vi "DiffDrivePoseEst2_Relative_Example.vi"() -> ()   [LabVIEW 2019]
doc: "This WebSockets API example VI acts as a server for an incoming websockets connection. Receives/sends string data to the connected client."
uses:
  <vilib>/Rock Robotics/WPI/ThirdParty/JAS_Junk/TrajLib/Trajectory_Library.lvlib
  <vilib>/Rock Robotics/WPI/ThirdParty/JAS_Junk/TrajLib/TypeDef/FieldDisp_ElementPicture.ctl
  <vilib>/Rock Robotics/WPI/ThirdParty/JAS_Junk/TrajLib/TypeDef/TRANSLATION2D.ctl
  <vilib>/Rock Robotics/WPI/ThirdParty/JAS_Junk/TrajLib/TypeDef/ROTATION2D.ctl
  <vilib>/Rock Robotics/WPI/ThirdParty/JAS_Junk/TrajLib/TypeDef/POSE2D.ctl
panel:
  in  "Ramsette\nAuto":bool=TRUE
  out "Odom Pose\n Ft, Deg":T1 {"ROTATION"."SIN" format="%13.4f"; "ROTATION"."COS" format="%13.4f"; "ROTATION"."VALUE" format="%13.4f"; "TRANSLATION"."Y" format="%14.3f"; "TRANSLATION"."X" format="%14.3f"}
  out "Trajectory\nAtReference":bool
  out "ROBOT":T4
  in  "Tab Control":T5(tab)
  out "Field Picture":picture
  out "Right Motor Dmd":dbl format="%20.3f"
  out "Left Motor Dmd":dbl format="%20.3f"
  out "Gyro Heading (Deg)":dbl format="%20.3f"
  out "Left Motor Dist (Ft)":dbl format="%20.3f"
  out "Right Motor Dist (Ft)":dbl format="%20.3f"
  out "Left Motor Vel - PV (Ft/Sec)":dbl format="%20.3f"
  out "Right Motor Vel - PV (Ft/Sec)":dbl format="%20.3f"
  out "Odometry sim abs\n Pose":T1={"TRANSLATION"={"X"=1.0, "Y"=1.0}, "ROTATION"={"VALUE"=0.0, "COS"=1.0, "SIN"=0.0}} {"ROTATION"."SIN" format="%13.4f"; "ROTATION"."COS" format="%13.4f"; "ROTATION"."VALUE" format="%13.4f"; "TRANSLATION"."Y" format="%14.3f"; "TRANSLATION"."X" format="%14.3f"}
  out "Trajectory Error":T6(graph)
  in  "Follow Relative\nTrajectory":bool
  in  "Spin Right":bool
  in  "Spin Left":bool
  in  "Reverse":bool
  in  "Forward":bool
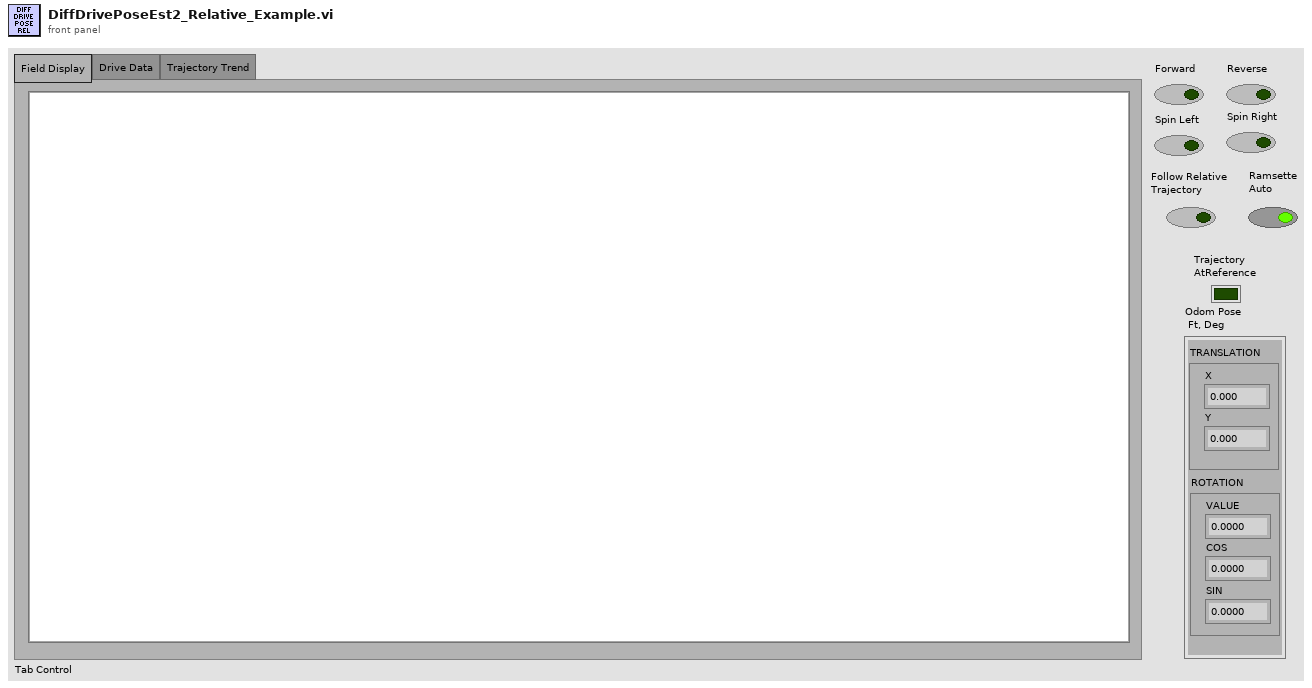
[diagram p1: front panel]
types:
  T1 = typedef "Trajectory_Library.lvlib/POSE2D.ctl" = cluster{"TRANSLATION":T2, "ROTATION":T3}
  T2 = typedef "Trajectory_Library.lvlib/TRANSLATION2D.ctl" = cluster{"X":dbl, "Y":dbl}
  T3 = typedef "Trajectory_Library.lvlib/ROTATION2D.ctl" = cluster{"VALUE":dbl, "COS":dbl, "SIN":dbl}
  T4 = typedef "Trajectory_Library.lvlib/FieldDisp_ElementPicture.ctl" = picture
  T5 = enum32{"Field Display", "Drive Data", "Trajectory Trend"}
  T6 = cluster{"Traj X Err Ft":dbl, "Traj Y Err Ft":dbl, "Traj Heading Err Deg":dbl, dbl}
  T7 = typedef "Trajectory_Library.lvlib/FieldDisp_FieldElement.ctl" = cluster{"ONE-8-bit pixmap":u8[][], "Two-Array":cdb[][], "Three-Numeric":i32, "Four-Numeric":i32, "Five-Numeric":cdb, "Six-colors":u32[], "Seven-new element/subarray":u32, "Left Poxel":dbl, "Top Pixel":dbl, "Width Pix/Ft":dbl, "Height Pix/Ft":dbl, "Element Picture Ref":refnum<vi>}
  T8 = typedef "Trajectory_Library.lvlib/TRAJECTORY.ctl" = cluster{"TotalTImeSecs":dbl, "States":T9[]}
  T9 = typedef "Trajectory_Library.lvlib/TRAJ_STATE.ctl" = cluster{"TimeSeconds":dbl, "Velocity":dbl, "Acceleration":dbl, "POSE":T1, "Curvature":dbl}
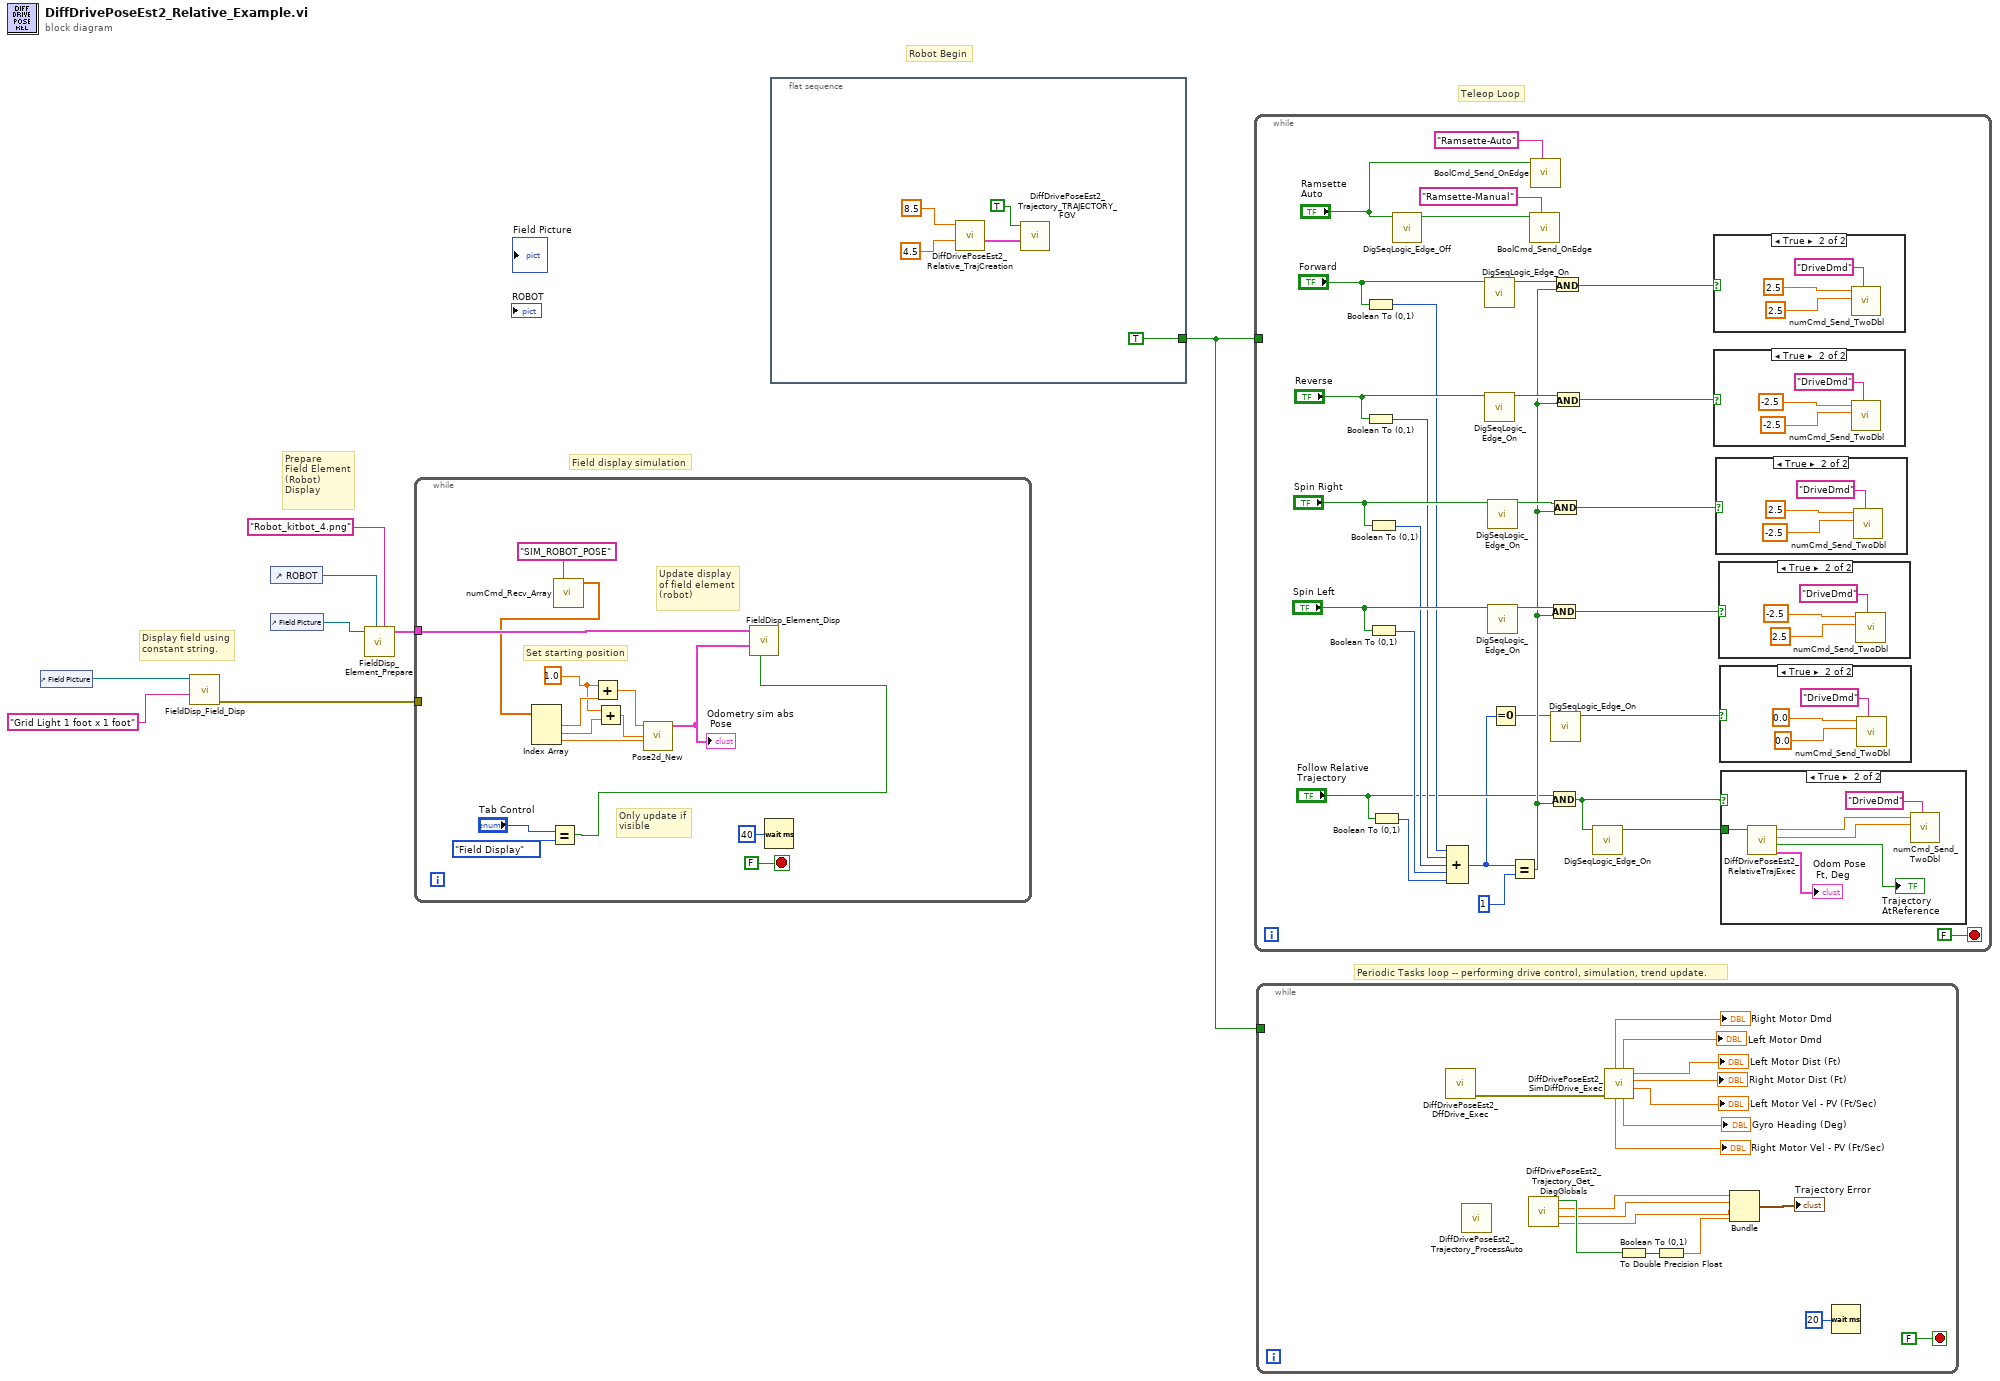
[diagram p0: block diagram]
diagram:
  # "Robot Begin"
  # "Periodic Tasks loop -- performing drive control, simulation, trend update."
  # "Field display simulation"
  # "Teleop Loop"
  # "Display field using\nconstant string."
  # "Prepare\nField Element\n(Robot)\nDisplay"
  n1 = control-ref of="Field Picture"() -> (w4:refnum<vi>)
  n2 = call <vilib>:"FieldDisp_Field_Disp.vi"("Field Selector"="Grid Light 1 foot x 1 foot", "Picture in"=w4) -> ("error out"=w2:errorcluster)  [unwired: 9 in]
  n3 = control-ref of="ROBOT"() -> (w7:refnum<vi>)
  n4 = control-ref of="Field Picture"() -> (w8:refnum<vi>)
  n5 = call <vilib>:"FieldDisp_Element_Prepare.vi"("Element File Name"="Robot_kitbot_4.png" ("Picture FIle Name"), "Element Picture Ref"=w7, "Field Picture Ref"=w8) -> ("Field Element Info"=w5:T7)  [unwired: 7 in, 1 out]
  n6 = while {
    tunnel: w5 -> [w21]
    tunnel: w2 -> [_]
    stop <- FALSE stop-if-true
    w10 = 1.0 ("x")
    # "Set starting position"
    # "Update display\nof field element\n(robot)"
    # "Only update if\nvisible"
    n7 = Equal?(x="Tab Control", y=T5."Field Display") -> (x = y?=w9:bool)
    n8 = call <vilib>:"numCmd_Recv_Array.vi"("Command Name"="SIM_ROBOT_POSE") -> ("Values"=w17:dbl[])  [unwired: 8 in, 2 out]
    n9 = Index Array(array=w17) -> (element #1=w11:dbl, element #2=w12:dbl, element #3=w16:dbl)  [unwired: 3 in]
    n10 = Add(x=w10, y=w11) -> (x+y=w13:dbl)
    n11 = Add(x=w10, y=w12) -> (x+y=w14:dbl)
    n12 = call <vilib>:"Pose2d_New.vi"("Heading"=w16, "Y"=w14, "X"=w13) -> ("out POSe"=w15:T1)  [unwired: 8 in]
    "Odometry sim abs\n Pose" <- w15
    n13 = call <vilib>:"FieldDisp_Element_Disp.vi"("Visible"=w9, "Element Pose"=w15, "Element Info"=w21) -> ()  [unwired: 9 in]
    n14 = Wait (ms)(milliseconds to wait=u32 40) -> ()  [unwired: 1 out]
  }
  n15 = flat-sequence {
    tunnel: [TRUE] -> w1
    frame #0 {
      n16 = call "DiffDrivePoseEst2_Relative_TrajCreation.vi"("Effective Track Width Ft"=4.5, "Max Velocity Ft/Sec"=8.5) -> ("Relative Trajectory"=w24:T8)  [unwired: 6 in, 3 out]
      n17 = call "DiffDrivePoseEst2_Trajectory_TRAJECTORY_FGV.vi"("inTRAJECTORY"=w24, "WRITE"=TRUE) -> ()  [unwired: 9 in, 1 out]
    }
  }
  n18 = while {
    tunnel: w1 -> [_]
    stop <- FALSE stop-if-true
    n19 = Boolean To (0,1)(Boolean="Forward") -> (0, 1=w50:i16)
    n20 = Boolean To (0,1)(Boolean="Reverse") -> (0, 1=w51:i16)
    n21 = Boolean To (0,1)(Boolean="Spin Right") -> (0, 1=w52:i16)
    n22 = Boolean To (0,1)(Boolean="Spin Left") -> (0, 1=w53:i16)
    n23 = Boolean To (0,1)(Boolean="Follow Relative\nTrajectory") -> (0, 1=w54:i16)
    n24 = call <vilib>:"DigSeqLogic_Edge_Off.vi"("Input"="Ramsette\nAuto") -> ("Off Edge"=w31:bool)  [unwired: 10 in]
    n25 = Compound Arithmetic op=ADD(w50, w51, w52, w53, w54) -> (w42:i16)
    n26 = call <vilib>:"DigSeqLogic_Edge_On.vi"("Input"="Forward") -> ("On Edge"=w48:bool)  [unwired: 10 in]
    n27 = call <vilib>:"DigSeqLogic_Edge_On.vi"("Input"="Reverse") -> ("On Edge"=w47:bool)  [unwired: 10 in]
    n28 = call <vilib>:"DigSeqLogic_Edge_On.vi"("Input"="Spin Right") -> ("On Edge"=w46:bool)  [unwired: 10 in]
    n29 = call <vilib>:"DigSeqLogic_Edge_On.vi"("Input"="Spin Left") -> ("On Edge"=w45:bool)  [unwired: 10 in]
    n30 = Equal To 0?(x=w42) -> (x = 0?=w41:bool)
    n31 = Equal?(x=w42, y=i16 1) -> (x = y?=w44:bool)
    n32 = call <vilib>:"BoolCmd_Send_OnEdge.vi"("Command Name"="Ramsette-Manual", "Value"=w31) -> ()  [unwired: 9 in, 1 out]
    n33 = call <vilib>:"BoolCmd_Send_OnEdge.vi"("Command Name"="Ramsette-Auto", "Value"="Ramsette\nAuto") -> ()  [unwired: 9 in, 1 out]
    n34 = And(x=w45, y=w44) -> (x .and. y?=w36:bool)
    n35 = And(x="Follow Relative\nTrajectory", y=w44) -> (x .and. y?=w35:bool)
    n36 = And(x=w46, y=w44) -> (x .and. y?=w38:bool)
    n37 = call <vilib>:"DigSeqLogic_Edge_On.vi"("Input"=w41) -> ("On Edge"=w37:bool)  [unwired: 10 in]
    n38 = And(x=w48, y=w44) -> (x .and. y?=w40:bool)
    n39 = And(x=w47, y=w44) -> (x .and. y?=w39:bool)
    n40 = call <vilib>:"DigSeqLogic_Edge_On.vi"("Input"=w35) -> ("On Edge"=w34:bool)  [unwired: 10 in]
    n41 = case shown="True" w40 {
      frame False {
      }
      frame True {
        n42 = call <vilib>:"numCmd_Send_TwoDbl.vi"("Command Name"="DriveDmd", "Value 2"=2.5, "Value 1"=2.5) -> ()  [unwired: 8 in, 1 out]
      }
    }
    n43 = case shown="True" w39 {
      frame False {
      }
      frame True {
        n44 = call <vilib>:"numCmd_Send_TwoDbl.vi"("Command Name"="DriveDmd", "Value 2"=-2.5, "Value 1"=-2.5) -> ()  [unwired: 8 in, 1 out]
      }
    }
    n45 = case shown="True" w38 {
      frame False {
      }
      frame True {
        n46 = call <vilib>:"numCmd_Send_TwoDbl.vi"("Command Name"="DriveDmd", "Value 2"=-2.5, "Value 1"=2.5) -> ()  [unwired: 8 in, 1 out]
      }
    }
    n47 = case shown="True" w36 {
      frame False {
      }
      frame True {
        n48 = call <vilib>:"numCmd_Send_TwoDbl.vi"("Command Name"="DriveDmd", "Value 2"=2.5, "Value 1"=-2.5) -> ()  [unwired: 8 in, 1 out]
      }
    }
    n49 = case shown="True" w37 {
      frame False {
      }
      frame True {
        n50 = call <vilib>:"numCmd_Send_TwoDbl.vi"("Command Name"="DriveDmd", "Value 2"=0.0, "Value 1"=0.0) -> ()  [unwired: 8 in, 1 out]
      }
    }
    n51 = case shown="True" w35 {
      tunnel: w34 -> [_ w60]
      frame False {
      }
      frame True {
        n52 = call "DiffDrivePoseEst2_RelativeTrajExec.vi"("Init"=w60) -> ("Odom Pose Eng"=→"Odom Pose\n Ft, Deg":T1, "AtReference"=→"Trajectory\nAtReference":bool, "Right Speed Target"=w62:dbl, "Left Speed Target"=w63:dbl)  [unwired: 7 in]
        n53 = call <vilib>:"numCmd_Send_TwoDbl.vi"("Command Name"="DriveDmd", "Value 2"=w62, "Value 1"=w63) -> ()  [unwired: 8 in, 1 out]
      }
    }
  }
  n54 = while {
    tunnel: w1 -> [_]
    stop <- FALSE stop-if-true
    n55 = call "DiffDrivePoseEst2_DffDrive_Exec.vi"() -> ("error out"=w87:errorcluster)  [unwired: 11 in]
    n56 = call "DiffDrivePoseEst2_Trajectory_ProcessAuto.vi"() -> ()  [unwired: 12 in]
    n57 = call "DiffDrivePoseEst2_Trajectory_Get_DiagGlobals.vi"() -> ("Traj Heading Err Deg"=w80:dbl, "Traj Y Err Ft"=w81:dbl, "Traj X Err Ft"=w82:dbl, "AtReference"=w84:bool)  [unwired: 8 in]
    n58 = call "DiffDrivePoseEst2_SimDiffDrive_Exec.vi"("error in (no error)"=w87) -> ("Left Motor Vel - PV (Ft/Sec)"=→"Left Motor Vel - PV (Ft/Sec)":dbl, "Right Motor Dist (Ft)"=→"Right Motor Dist (Ft)":dbl, "Left Motor Dist (Ft)"=→"Left Motor Dist (Ft)":dbl, "Gyro Heading (Deg)"=→"Gyro Heading (Deg)":dbl, "Left Motor Dmd"=→"Left Motor Dmd":dbl, "Right Motor Vel - PV (Ft/Sec)"=→"Right Motor Vel - PV (Ft/Sec)":dbl, "Right Motor Dmd"=→"Right Motor Dmd":dbl)  [unwired: 3 in, 1 out]
    n59 = Boolean To (0,1)(Boolean=w84) -> (0, 1=w85:i16)
    n60 = To Double Precision Float(number=w85) -> (double precision float=w83:dbl)
    n61 = Bundle("Traj X Err Ft"=w82, "Traj Y Err Ft"=w81, "Traj Heading Err Deg"=w80, w83) -> (→"Trajectory Error":T6)  [unwired: 1 in]
    n62 = Wait (ms)(milliseconds to wait=u32 20) -> ()  [unwired: 1 out]
  }
